vi "FloatApprox.vi"(2 "y":dbl, 3 "x":dbl) -> (0 "x ~ y?":bool)   [LabVIEW 2016]
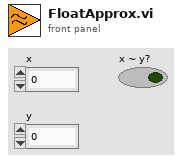
[diagram p1: front panel]
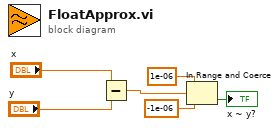
[diagram p0: block diagram]
diagram:
  n1 = Subtract(x="x", y="y") -> (x-y=w3:dbl)
  n2 = In Range and Coerce(upper limit=1e-06, x=w3, lower limit=-1e-06 ("upper limit")) -> (In Range?=→"x ~ y?":bool)  [unwired: 1 out]
